vi "Open.vi"(8 "error in":errorcluster, 9 "timeout (-1)":i32=-1, 11 "Engine Runtime Interface in":refnum<class "Engine Runtime Interface.lvclass">) -> (0 "error out":errorcluster, 3 "Engine Runtime Interface out":refnum<class "Engine Runtime Interface.lvclass">)   [LabVIEW 2014, in "Engine Runtime Interface.lvclass"]
doc: "This function initializes the engine process and gets it in a state where it is ready to accept a configuration."
uses:
  Engine Runtime Interface.lvclass
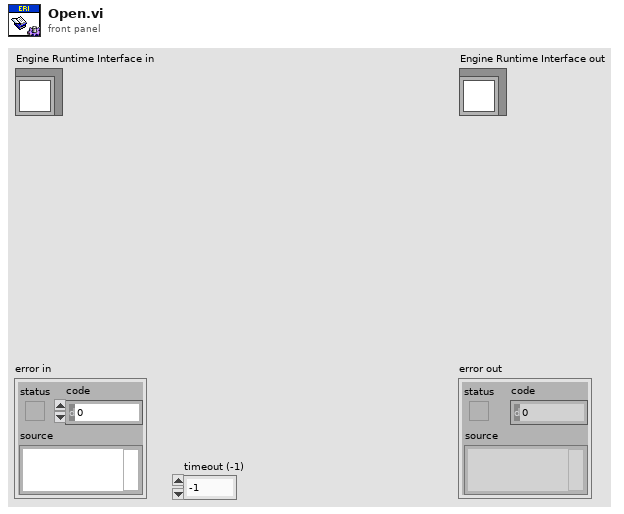
[diagram p1: front panel]
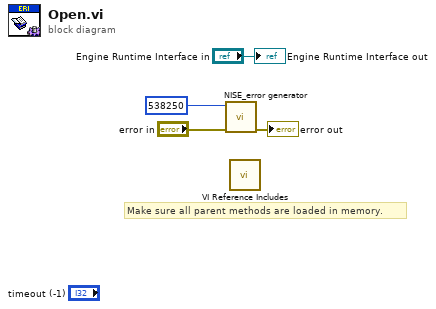
[diagram p0: block diagram]
diagram:
  # "Make sure all parent methods are loaded in memory."
  n1 = call <vilib>:"NISE_error generator.vi"("error in"="error in", "error code (0)"=538250) -> ("error out"=→"error out":errorcluster)  [unwired: 7 in]
  n2 = call "VI Reference Includes.vi"() -> ()  [unwired: 12 in]
  "Engine Runtime Interface out" <- "Engine Runtime Interface in"
